vi "Kafka_GetMinMaxOffsets.vi"(8 "error in (no error)":errorcluster, 11 "Consumer Handle":string) -> (0 "error out":errorcluster, 1 "Min Offset":i64, 2 "Max Offset":i64, 3 "Consumer Handle":string)   [LabVIEW 2019]
uses:
  VS2017/KafkaLVLib/x64/Debug/KafkaLVLib.dll
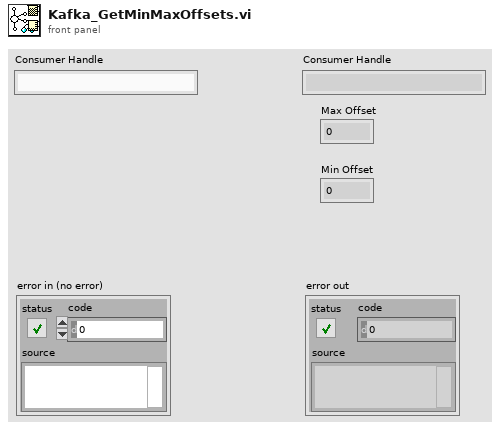
[diagram p1: front panel]
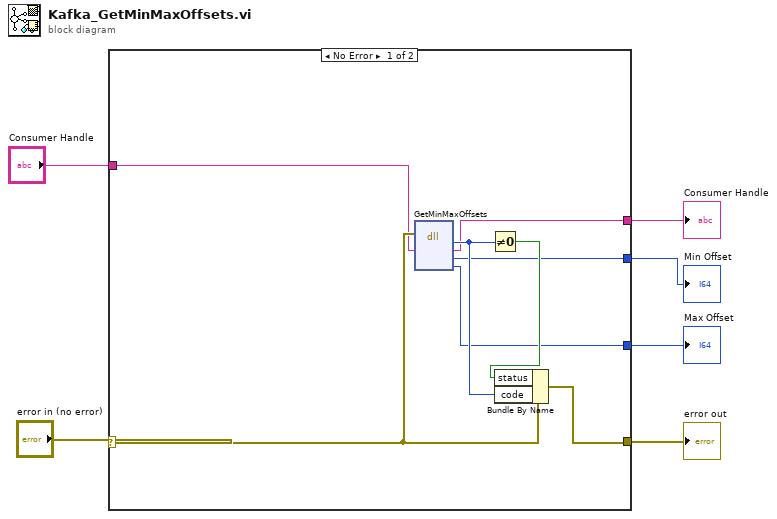
[diagram p0: block diagram]
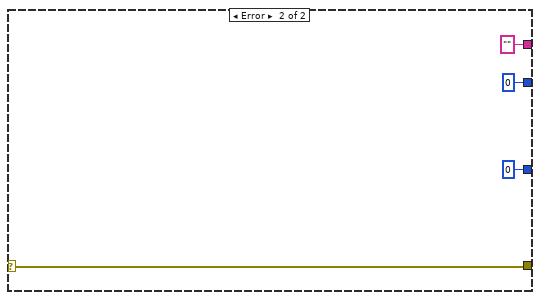
[diagram p2: hidden frame]
diagram:
  n1 = case shown="No Error" "error in (no error)" {
    selector: "error in (no error)" -> [w11 w17]
    tunnel: [w12 w17] -> w5
    tunnel: [w7 "" ("consumerHandle")] -> w4
    tunnel: "Consumer Handle" -> [w10 _]
    tunnel: [w9 i64 0 ("minOffset")] -> w2
    tunnel: [w8 i64 0 ("maxOffset")] -> w1
    frame No Error {
      n2 = dll-call lib="C:/Users/schandho/OneDrive - National Instruments/Research/Virtualization/SemiADV/KafkaLVLib/VS2017/KafkaLVLib/x64/Debug/KafkaLVLib.dll" fn="GetMinMaxOffsets"(error in=w11, "consumerHandle"=w10) -> ("error"=w13:i32, "consumerHandle"=w7:string, "minOffset"=w9:i64, "maxOffset"=w8:i64)  [unwired: 4 in, 2 out]
      n3 = Not Equal To 0?(x=w13) -> (x != 0?=w14:bool)
      n4 = Bundle By Name(cluster=w11, "status"=w14, "code"=w13) -> (w12:errorcluster)
    }
    frame Error {
    }
  }
  "error out" <- w5
  "Consumer Handle" <- w4
  "Min Offset" <- w2
  "Max Offset" <- w1
